vi "singleRequest.vi"(9 "RequestId":i32, 10 "Debug":bool, 11 "httpRequestID":u32) -> ()   [LabVIEW 2014]
uses:
  FRCts20_EspEngine.lvlib
  <vilib>/wsapi/NI_WebServices.lvlib
  <vilib>/wsapi/subVIs/Set Boolean ESP Variable.vi
  Backend/source/VI Source/FRCts20_Backend_API/FRCts20_Backend_API_Status.ctl
  Backend/source/VI Source/FRCts20_Backend_API/FRCts20_Backend_API.lvlib
  Web Methods/source/VI Source/Web Method Public Interface/FRCts20_WebMethods_ctl_request.ctl
  Web Methods/source/VI Source/FRCts20_WebMethods.lvlib
  Web Methods/source/VI Source/Web Method Public Interface/FRCts20_WebMethods_ctl_teamIdentifier.ctl
  Backend/source/VI Source/FRCts20_Backend_API/FRCts20_Backend_API_SW.ctl
  Web Methods/source/VI Source/Web Method Public Interface/FRCts20_WebMethods_ctl_singleTeam.ctl
  TypeDefs/FRCts20_EspEngine_Team.ctl
panel:
  in  "Team":T1={"Team"={"Events"=[], "Robot Name"="", "Kinect"=FALSE, "Vision"=FALSE, "Can"=FALSE, "Tags"="", "Avatar URL"="", "Team"={"Team Nickname"="", "Team Number "=22, "UniqueId"=2}, "SWType"=""}, "RequestListLength"=3, "Requests"=[{"Event"="", "Description"="", "Status"=enum."Open", "Open Date"="", "Last Update"="", "Close Date"="", "UniqueId"=0, "Team"={"Team Nickname"="", "Team Number "=0, "UniqueId"=0}, "Comments"=[]}, {"Event"="", "Description"="", "Status"=enum."Open", "Open Date"="", "Last Update"="", "Close Date"="", "UniqueId"=0, "Team"={"Team Nickname"="", "Team Number "=0, "UniqueId"=0}, "Comments"=[]}, {"Event"="", "Description"="", "Status"=enum."Open", "Open Date"="", "Last Update"="", "Close Date"="", "UniqueId"=0, "Team"={"Team Nickname"="", "Team Number "=0, "UniqueId"=0}, "Comments"=[]}]}
  in  "Request":T5={"Event"="", "Description"="", "Status"=enum."Open", "Open Date"="", "Last Update"="", "Close Date"="", "UniqueId"=0, "Team"={"Team Nickname"="", "Team Number "=0, "UniqueId"=0}, "Comments"=[{"Request Number"=1.0, "Text"="", "Author"="Mark", "IsSolution"=FALSE, "Team"={"Team Nickname"="", "Team Identifier "=0.0}, "UniqueId"=1}, {"Request Number"=2.0, "Text"="", "Author"="Makr ", "IsSolution"=TRUE, "Team"={"Team Nickname"="", "Team Identifier "=0.0}, "UniqueId"=2}]}
  out "error out":errorcluster
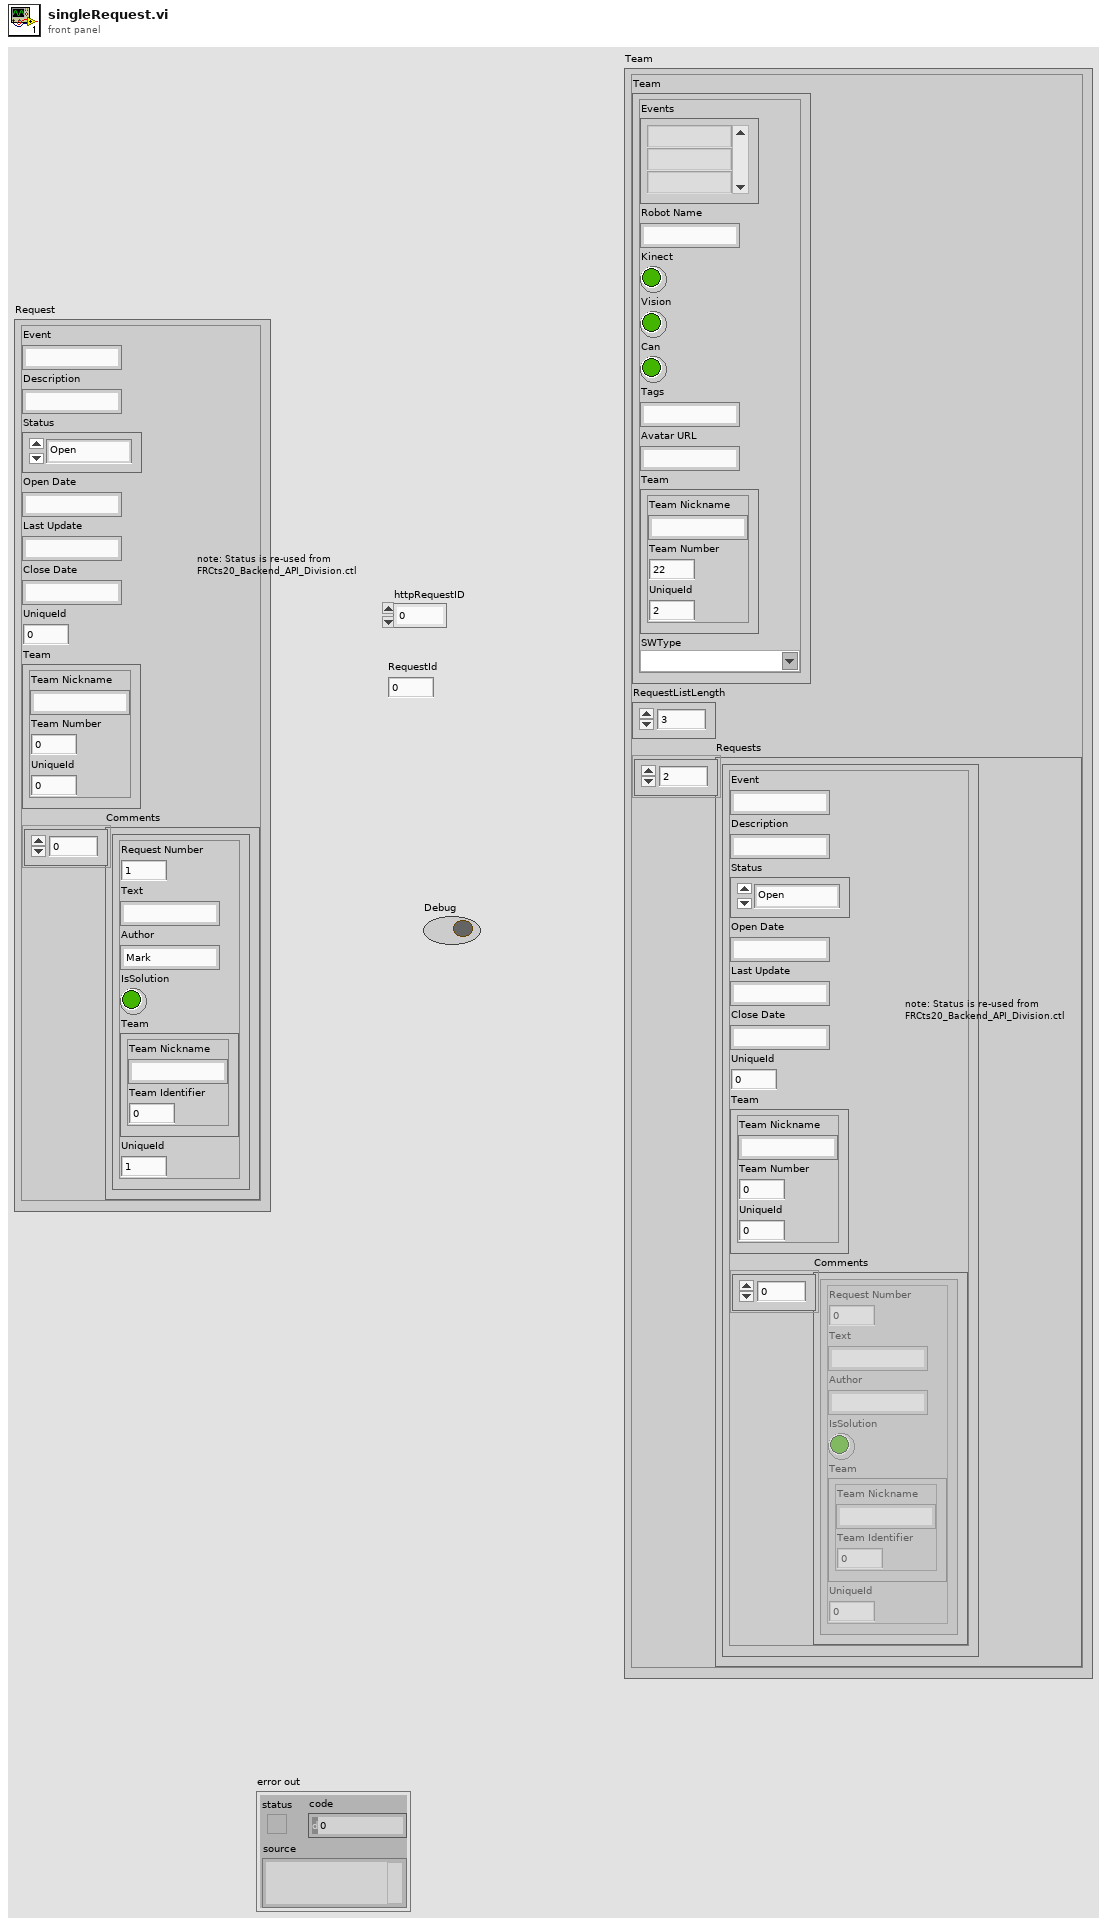
[diagram p1: front panel]
types:
  T1 = typedef "FRCts20_EspEngine.lvlib/FRCts20_EspEngine_Team.ctl" = cluster{"Team":T2, "RequestListLength":i16, "Requests":T5[]}
  T2 = typedef "FRCts20_WebMethods.lvlib/FRCts20_WebMethods_ctl_singleTeam.ctl" = cluster{"Events":string[], "Robot Name":string, "Kinect":bool, "Vision":bool, "Can":bool, "Tags":string, "Avatar URL":string, "Team":T3, "SWType":T4}
  T3 = typedef "FRCts20_WebMethods.lvlib/FRCts20_WebMethods_ctl_teamIdentifier.ctl" = cluster{"Team Nickname":string, "Team Number ":u32, "UniqueId":u32}
  T4 = typedef "FRCts20_Backend_API.lvlib/FRCts20_Backend_API_SW.ctl" = string
  T5 = typedef "FRCts20_WebMethods.lvlib/FRCts20_WebMethods_ctl_request.ctl" = cluster{"Event":string, "Description":string, "Status":T6, "Open Date":string, "Last Update":string, "Close Date":string, "UniqueId":i32, "Team":cluster{"Team Nickname":string, "Team Number ":i32, "UniqueId":i32}, "Comments":cluster{"Request Number":dbl, "Text":string, "Author":string, "IsSolution":bool, "Team":cluster{"Team Nickname":string, "Team Identifier ":dbl}, "UniqueId":i32}[]}
  T6 = typedef "FRCts20_Backend_API.lvlib/FRCts20_Backend_API_Status.ctl" = enum16{"Open", "In Work", "Closed"}
  T7 = typedef "FRCts20_EspEngine.lvlib/FRCts20_EspEngine_SearchBrowser.ctl" = cluster{"Event":cluster{"Event Index":u32, "Event Name":string, "Start Time":timestamp, "End Time":timestamp, "OpenIssues":u8, "IsLive":bool}[], "select-choice-software":string, "select-choice-location":string}
  T8 = typedef "FRCts20_EspEngine.lvlib/FRCts20_EspEngine_Request.ctl" = cluster{"Request":T5, "CommentListLength":i16}
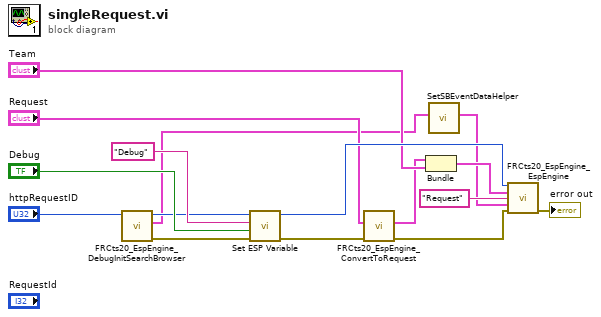
[diagram p0: block diagram]
diagram:
  n1 = call "FRCts20_EspEngine_DebugInitSearchBrowser.vi"("httpRequestID"="httpRequestID") -> ("error out"=w3:errorcluster, "SearchBrowser"=w2:T7, "httpRequestID out"=w4:u32)  [unwired: 8 in]
  n2 = call-poly <vilib>:"Set ESP Variable.vi"("error in (no error)"=w3, "value"="Debug", "key"="Debug", "httpRequestID"=w4) -> ("error out"=w11:errorcluster, "httpRequestID out"=w14:u32)  [unwired: 6 in]
  n3 = call "FRCts20_EspEngine_ConvertToRequest.vi"("error in (no error)"=w11, "Request"="Request") -> ("error out"=w10:errorcluster, "Request"=w7:T8)  [unwired: 8 in]
  n4 = Bundle("Request"=w7, "Team"="Team") -> (w6:cluster{"Request":T8, "Team":T1})  [unwired: 1 in]
  n5 = call "SetSBEventDataHelper.vi"("SearchBrowser"=w2) -> ("SearchBrowser"=w1:T7)  [unwired: 10 in]
  n6 = call "FRCts20_EspEngine_EspEngine.vi"("httpRequestID"=w14, "Cluster"=w6, "Page"="Request", "SearchBrowser"=w1, "error in (no error)"=w10) -> ("error out"=→"error out":errorcluster)  [unwired: 9 in, 1 out]
